vi "3.1-Joystick Behavior.vi"   [LabVIEW 2010]
uses:
  3.0 Flow Control/3.0 List of Loops.ctl
  4-High Neurons/4.1.2-Act Neuron TD.ctl
  3.0-Global.vi
  <vilib>/gmath/statdist.llb/Normal PDF.vi
  <vilib>/gmath/NI_Gmath.lvlib
types:
  T1 = typedef "3.0 List of Loops.ctl" = enum16{"3.0 State Update", "3.0 GUI", "3.1 Act", "3.1 4.7.1 Act UDP", "3.1 Joystick", "3.2 Where", "3.2.0 Kalman Filter", "3.2 4.7.2 Where UDP", "3.3 What", "3.3 4.7.3 What UDP", "3.4 How", "3.4 4.7.4 How UDP", "3.5 Limbic", "3.8 TCP", "3.6 Cerebellum", "3.8 TCP Act"}
  T2 = typedef "4.1.2-Act Neuron TD.ctl" = cluster{"Speed By Path":sgl[]}
  T3 = enum16{"Set Joystick", "Read Joystick", "Set Forebrain", "Read Forebrain", "Set Limbic", "Read Limbic", "Set Cerebellum", "Read Cerebellum", "Set Arbitrated", "Read Arbitrated", "Set LIDAR", "Read LIDAR"}
  T4 = typedef "4.1-Act Control Typedef.ctl" = cluster{"E-Stop":bool, "Restart":bool, "Extended Joystick":bool, "Begin":bool, "Time":i32, "Shutdown":bool, "Saitek Controler":T5, "Joystick Valid":bool}
  T5 = typedef "6.1-UDP Saitek.ctl" = cluster{"Stop":bool, "Setpoint":bool, "Run":bool, "Restart":bool, "Shutdown":bool, "Joystick\nMode 1":bool, "Joystick\nMode 2":bool, "Joystick \nMode 3":bool, "Joystick Mode 4":bool, "10":bool, "11":bool, "Pitch":sgl, "Roll":sgl, "Yaw":sgl, "Left":sgl, "Right":sgl}
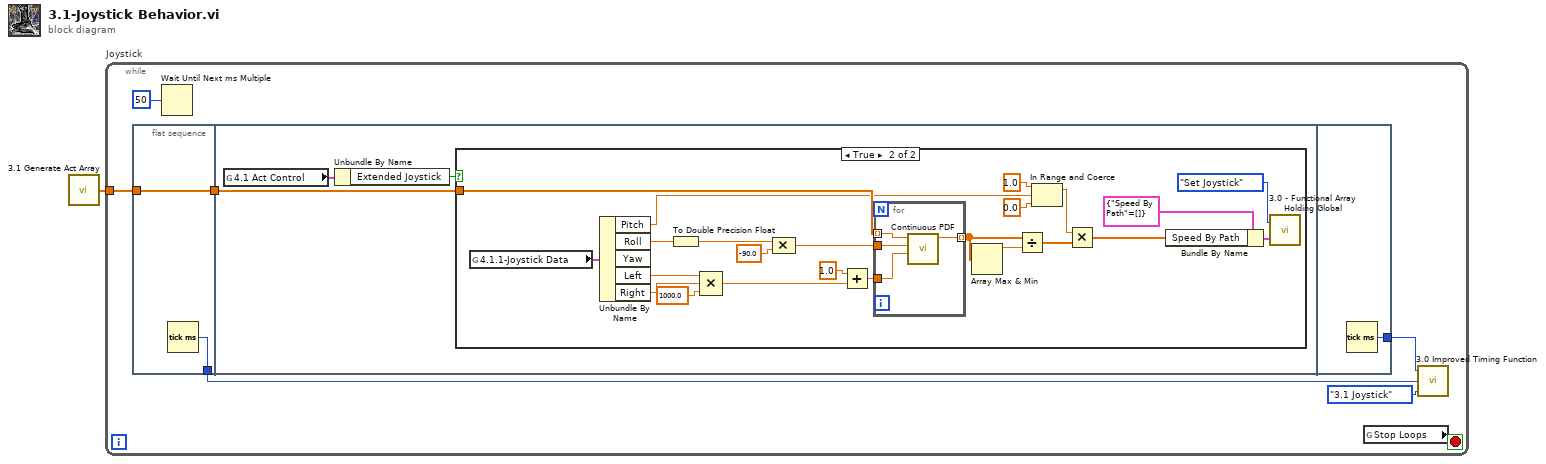
[diagram p0: block diagram]
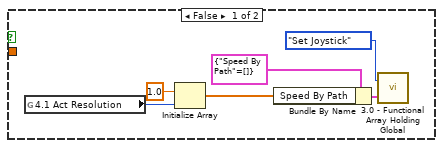
[diagram p2: hidden frame]
diagram:
  n1 = call "3.1 Generate Act Array.vi"() -> ("Array"=w1:dbl[])
  n2 = while "Joystick" {
    tunnel: w1 -> [w8]
    stop <- w7 stop-if-true
    n3 = flat-sequence {
      tunnel: w8 -> [w10]
      tunnel: [w10] -> w5
      tunnel: [w9] -> w3
      tunnel: w5 -> [w13]
      tunnel: [w47] -> w4
      frame #0 {
        n4 = Tick Count (ms)() -> (millisecond timer value=w9:u32)
      }
      frame #1 {
        n5 = global read "3.0-Global.vi" "4.1 Act Control"() -> (w12:T4)
        n6 = Unbundle By Name(w12) -> ("Extended Joystick"=w11:bool)
        n7 = case shown="True" w11 {
          tunnel: w13 -> [_ w40]
          frame False {
            n8 = global read "3.0-Global.vi" "4.1 Act Resolution"() -> (w14:u32)
            n9 = Initialize Array(1.0 ("element"), w14) -> (w16:dbl[])
            n10 = Bundle By Name(cluster=T2 {"Speed By Path"=[]} ("Input Act Neurons"), "Speed By Path"=w16) -> (w17:T2)
            n11 = call "3.0 - Functional Array Holding Global.vi"("Input Act Neurons"=w17, "Mode"=T3."Set Joystick") -> ()  [unwired: 1 out]
          }
          frame True {
            n12 = global read "3.0-Global.vi" "4.1.1-Joystick Data"() -> (w42:T5)
            n13 = Unbundle By Name(w42) -> ("Pitch"=w24:sgl, "Roll"=w41:sgl, "Left"=w28:sgl, "Right"=w29:sgl)  [unwired: 1 out]
            n14 = To Double Precision Float(number=w41) -> (double precision float=w35:dbl)
            n15 = Compound Arithmetic op=MULTIPLY(w28, w29, 1000.0) -> (w33:dbl)
            n16 = Compound Arithmetic op=MULTIPLY(w35, -90.0 ("value")) -> (w34:dbl)
            n17 = Add(x=1.0, y=w33) -> (x+y=w27:dbl)
            n18 = for {
              tunnel: w27 -> [w46]
              tunnel: w34 -> [w45]
              tunnel: w40 -> [w44] mode=indexing
              tunnel: [w43] -> w32 mode=indexing
              n19 = call-poly <vilib>:"Continuous PDF.vi"("std"=w46, "mean"=w45, "x"=w44) -> ("pdf(x)"=w43:dbl)  [unwired: 7 in, 1 out]
            }
            n20 = Array Max & Min(array=w32) -> (max value=w31:dbl)  [unwired: 3 out]
            n21 = Divide(x=w32, y=w31) -> (x/y=w30:dbl[])
            n22 = In Range and Coerce(upper limit=sgl 1.0, x=w24, lower limit=sgl 0.0) -> (coerced(x)=w23:sgl)  [unwired: 1 out]
            n23 = Multiply(x=w23, y=w30) -> (x*y=w25:dbl[])
            n24 = Bundle By Name(cluster=T2 {"Speed By Path"=[]} ("Forebrain Act Neurons"), "Speed By Path"=w25) -> (w37:T2)
            n25 = call "3.0 - Functional Array Holding Global.vi"("Input Act Neurons"=w37, "Mode"=T3."Set Joystick") -> ()  [unwired: 1 out]
          }
        }
      }
      frame #2 {
        n26 = Tick Count (ms)() -> (millisecond timer value=w47:u32)
      }
    }
    n27 = Wait Until Next ms Multiple(millisecond multiple=u32 50) -> ()  [unwired: 1 out]
    n28 = global read "3.0-Global.vi" "Stop Loops"() -> (w7:bool)
    n29 = call "3.0 Improved Timing Function.vi"("Loop"=3.0_List_of_Loops."3.1 Joystick", "Start"=w3, "End"=w4) -> ()  [unwired: 1 in]
  }
